vi "Write status code.vi"(8 "error in (no error)":errorcluster, 10 "status code":u16, 11 "httpRequest in":refnum<class "httpResponse.lvclass">) -> (0 "error out":errorcluster, 3 "httpRequest out":refnum<class "httpResponse.lvclass">)   [LabVIEW 2020]
uses:
  httpResponse.lvclass
  httpResponse.lvclass/httpResponse.ctl
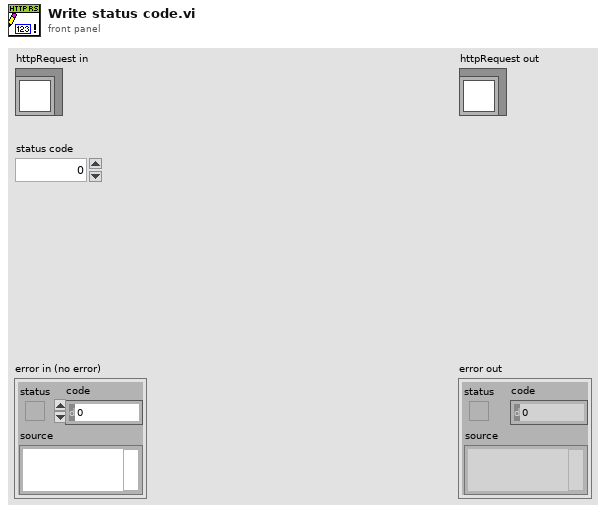
[diagram p1: front panel]
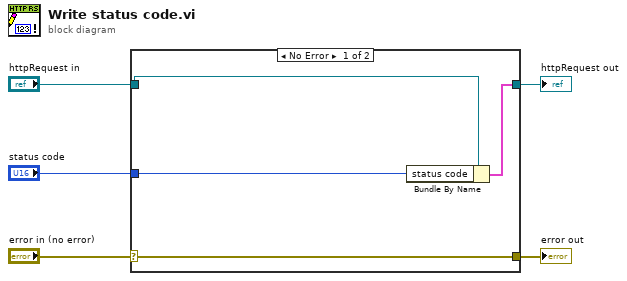
[diagram p0: block diagram]
diagram:
  n1 = case shown="No Error" "error in (no error)" {
    selector: "error in (no error)" -> [w9 w10]
    tunnel: [w9 w10] -> w4
    tunnel: [w7 w11] -> w2
    tunnel: "httpRequest in" -> [w8 w11]
    tunnel: "status code" -> [w6 _]
    frame No Error {
      n2 = Bundle By Name(cluster=w8, "status code"=w6) -> (w7:cluster{})
    }
    frame Error {
    }
  }
  "error out" <- w4
  "httpRequest out" <- w2
